vi "Day 04 Part 1.vi"(11 "Input":string) -> (3 "Output":u32)   [LabVIEW 2021]
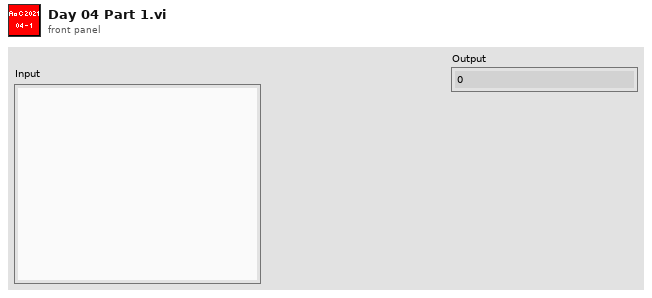
[diagram p1: front panel]
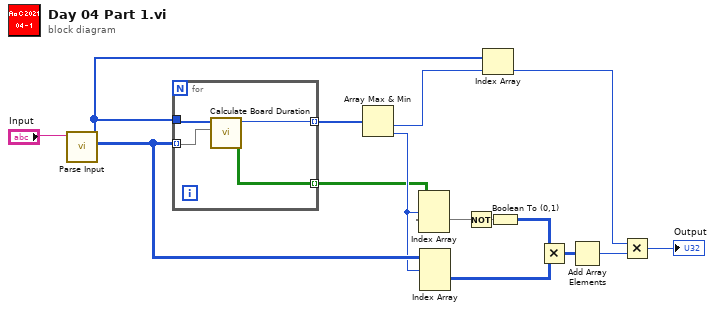
[diagram p0: block diagram]
diagram:
  n1 = call "Parse Input.vi"("Input"="Input") -> ("Boards"=w13:i32[][][], "Draw"=w1:i32[])  [unwired: 9 in]
  n2 = for {
    tunnel: w13 -> [w18] mode=indexing
    tunnel: w1 -> [w19]
    tunnel: [w17] -> w14 mode=indexing
    tunnel: [w16] -> w8 mode=indexing
    n3 = call "Calculate Board Duration.vi"("Board"=w18, "Draw"=w19) -> ("Marked"=w16:bool[][], "Duration"=w17:i32)  [unwired: 6 in, 2 out]
  }
  n4 = Array Max & Min(array=w14) -> (min value=w10:i32, min index (indices)=w12:i32)  [unwired: 2 out]
  n5 = Index Array(array=w8, index (dim 0)=w12) -> (element=w7:bool[][])  [unwired: 2 in]
  n6 = Index Array(array=w13, index (dim 0)=w12) -> (element=w5:i32[][])  [unwired: 2 in]
  n7 = Not(x=w7) -> (.not. x?=w6:bool[][])
  n8 = Index Array(array=w1, index=w10) -> (element=w9:i32)
  n9 = Boolean To (0,1)(Boolean=w6) -> (0, 1=w4:i16[][])
  n10 = Multiply(x=w4, y=w5) -> (x*y=w3:i32[][])
  n11 = Add Array Elements(numeric array=w3) -> (sum=w2:i32)
  n12 = Multiply(x=w9, y=w2) -> (x*y=→"Output":i32)
